vi "computeDistance.vi"(3 "Array":dbl[][](array[numeric]), 4 "Position":T1, 5 "String":string) -> (0 "1":bool, 1 "2":bool, 2 "distance":dbl)   [LabVIEW 2014]
uses:
  <vilib>/Utility/miscctls.llb/LVPositionTypeDef.ctl
panel:
  # "要走幾格不是幾單位"
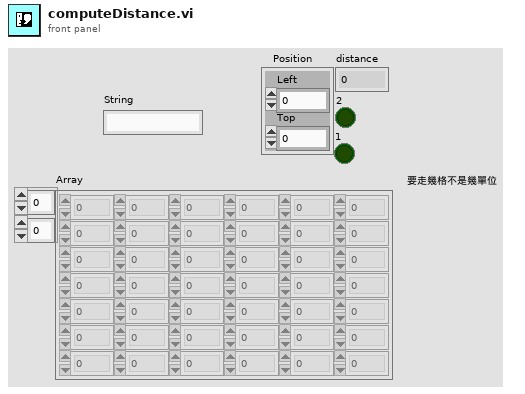
[diagram p1: front panel]
types:
  T1 = typedef "LVPositionTypeDef.ctl" = cluster{"Left":i32, "Top":i32}
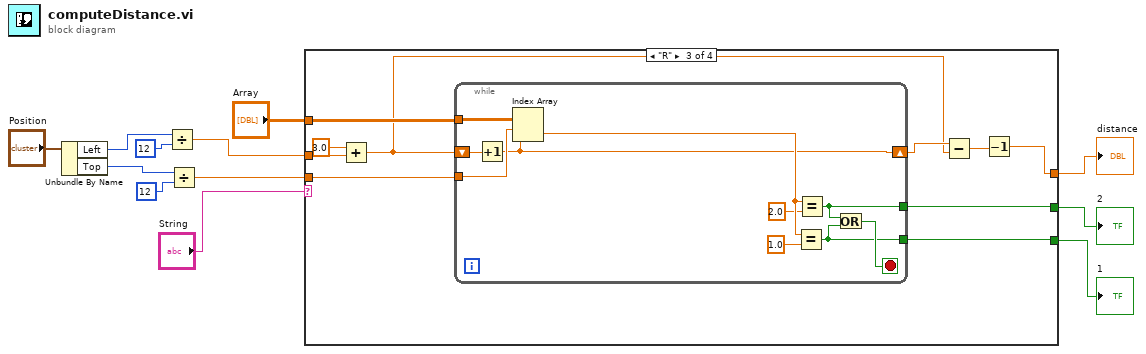
[diagram p0: block diagram]
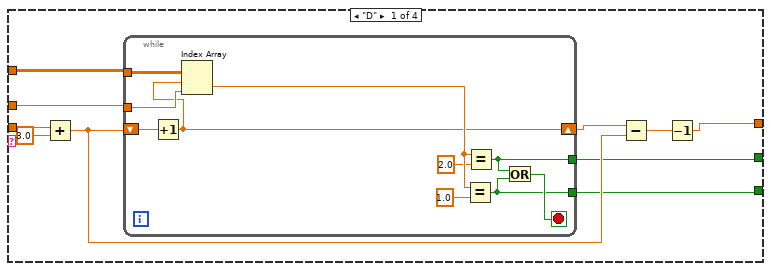
[diagram p2: hidden frame]
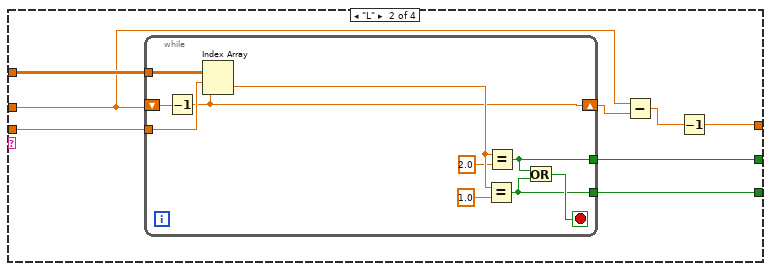
[diagram p3: hidden frame]
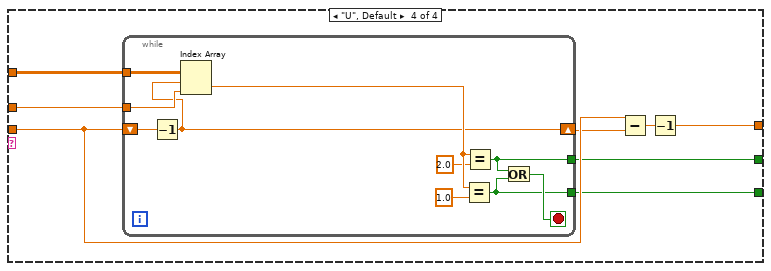
[diagram p4: hidden frame]
diagram:
  n1 = Unbundle By Name("Position") -> ("Left"=w11:i32, "Top"=w10:i32)
  n2 = Divide(x=w11, y=12) -> (x/y=w4:dbl)
  n3 = Divide(x=w10, y=12) -> (x/y=w5:dbl)
  n4 = case shown="\"R\"" "String" {
    tunnel: "Array" -> [w19 w40 w58 w78]
    tunnel: w5 -> [w22 w39 w57 w76]
    tunnel: w4 -> [w20 w38 w60 w77]
    tunnel: [w15 w35 w53 w73] -> w3
    tunnel: [w14 w34 w52 w72] -> w2
    tunnel: [w13 w33 w51 w71] -> w1
    frame "D" {
      n5 = Add(x=w22, y=3.0) -> (x+y=w17:dbl)
      n6 = while {
        tunnel: w19 -> [w32]
        tunnel: w20 -> [w31]
        shift-right: [w25] -> w18
        shift-left: w17 -> [w26]
        tunnel: [w24] -> w14
        tunnel: [w23] -> w13
        stop <- w27 stop-if-true
        n7 = Increment(x=w26) -> (x+1=w25:dbl)
        n8 = Index Array(array=w32, index (row)=w25, index (col)=w31) -> (element=w29:dbl)
        n9 = Equal?(x=w29, y=1.0) -> (x = y?=w23:bool)
        n10 = Equal?(x=w29, y=2.0) -> (x = y?=w24:bool)
        n11 = Or(x=w24, y=w23) -> (x .or. y?=w27:bool)
      }
      n12 = Subtract(x=w18, y=w17) -> (x-y=w16:dbl)
      n13 = Decrement(x=w16) -> (x-1=w15:dbl)
    }
    frame "L" {
      n14 = while {
        tunnel: w40 -> [w50]
        shift-right: [w41] -> w37
        shift-left: w38 -> [w42]
        tunnel: [w45] -> w34
        tunnel: [w44] -> w33
        tunnel: w39 -> [w43]
        stop <- w46 stop-if-true
        n15 = Decrement(x=w42) -> (x-1=w41:dbl)
        n16 = Index Array(array=w50, index (row)=w43, index (col)=w41) -> (element=w48:dbl)
        n17 = Equal?(x=w48, y=1.0) -> (x = y?=w44:bool)
        n18 = Equal?(x=w48, y=2.0) -> (x = y?=w45:bool)
        n19 = Or(x=w45, y=w44) -> (x .or. y?=w46:bool)
      }
      n20 = Subtract(x=w38, y=w37) -> (x-y=w36:dbl)
      n21 = Decrement(x=w36) -> (x-1=w35:dbl)
    }
    frame "R" {
      n22 = Add(x=3.0, y=w60) -> (x+y=w55:dbl)
      n23 = while {
        tunnel: w58 -> [w70]
        shift-right: [w61] -> w56
        shift-left: w55 -> [w62]
        tunnel: [w65] -> w52
        tunnel: [w64] -> w51
        tunnel: w57 -> [w63]
        stop <- w66 stop-if-true
        n24 = Increment(x=w62) -> (x+1=w61:dbl)
        n25 = Index Array(array=w70, index (row)=w63, index (col)=w61) -> (element=w68:dbl)
        n26 = Equal?(x=w68, y=1.0) -> (x = y?=w64:bool)
        n27 = Equal?(x=w68, y=2.0) -> (x = y?=w65:bool)
        n28 = Or(x=w65, y=w64) -> (x .or. y?=w66:bool)
      }
      n29 = Subtract(x=w56, y=w55) -> (x-y=w54:dbl)
      n30 = Decrement(x=w54) -> (x-1=w53:dbl)
    }
    frame "U", Default {
      n31 = while {
        tunnel: w78 -> [w88]
        tunnel: w77 -> [w87]
        shift-right: [w81] -> w74
        shift-left: w76 -> [w82]
        tunnel: [w80] -> w72
        tunnel: [w79] -> w71
        stop <- w83 stop-if-true
        n32 = Decrement(x=w82) -> (x-1=w81:dbl)
        n33 = Index Array(array=w88, index (row)=w81, index (col)=w87) -> (element=w85:dbl)
        n34 = Equal?(x=w85, y=1.0) -> (x = y?=w79:bool)
        n35 = Equal?(x=w85, y=2.0) -> (x = y?=w80:bool)
        n36 = Or(x=w80, y=w79) -> (x .or. y?=w83:bool)
      }
      n37 = Subtract(x=w76, y=w74) -> (x-y=w75:dbl)
      n38 = Decrement(x=w75) -> (x-1=w73:dbl)
    }
  }
  "distance" <- w3
  "2" <- w2
  "1" <- w1
